vi "AverageSubVIMarcoGonzalez.vi"(1 "z":dbl, 2 "y":dbl, 3 "x":dbl) -> (0 "A":dbl)   [LabVIEW 2012]
doc: "This Sub VI will calculate the average of three numbers."
panel:
  # "Marco Gonzalez\nEA 3\n02/21/2017"
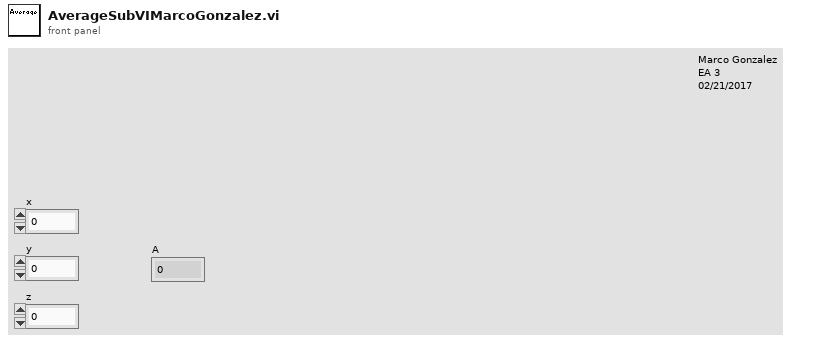
[diagram p1: front panel]
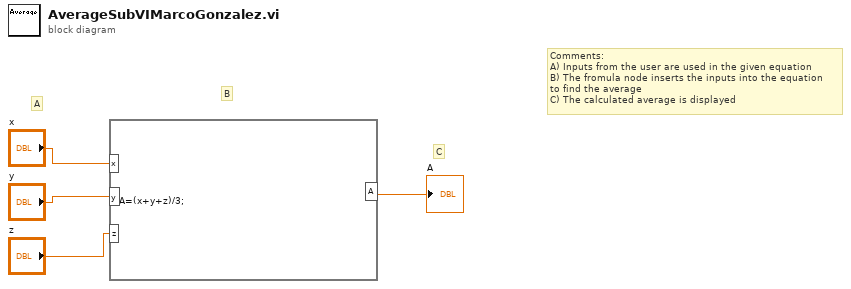
[diagram p0: block diagram]
diagram:
  # "C"
  # "A"
  # "B"
  # "Comments:\nA) Inputs from the user are used in the given equation\nB) The fromula node inserts the inputs into the equation\nto find the average\nC) The calculated average is displayed"
  n1 = formula code="A=(x+y+z)/3;"("x"="x", "y"="y", "z"="z") -> ("A"=→"A":dbl)
